vi "Idle_WeatherStationComms.vi"(0 "VISA in":refnum<visa-resource-name>="LuftWS", 5 "WS_Commands":enum16{"OpenWS", "ReadTRHP", "CloseWS"}(ring)=enum."ReadTRHP", 7 "wait (ms)":u32=50, 11 "Error In":errorcluster) -> (4 "VISA out":refnum<visa-resource-name>="LuftWS", 6 "TRHP":T1={"Temp"=27.834401709401718, "RelH"=23.501221001221, "Press"=837.9120879120879, "AbH"=6.333943833943834}, 8 "StringResponse":string, 15 "Error Out":errorcluster)   [LabVIEW 2012]
uses:
  WVD-MCSupdate/WVDNewArchitectureUpdate/WVD_Architecture_Update/WVDIAL_GlobalVariables.vi
  <vilib>/Instr/_visa.llb/VISA Configure Serial Port (Instr).vi
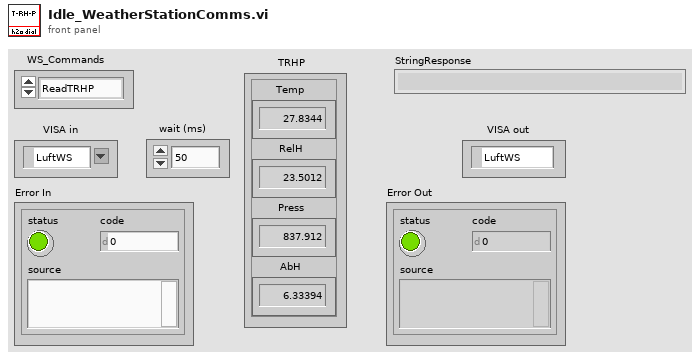
[diagram p1: front panel]
types:
  T1 = cluster{"Temp":dbl, "RelH":dbl, "Press":dbl, "AbH":dbl}
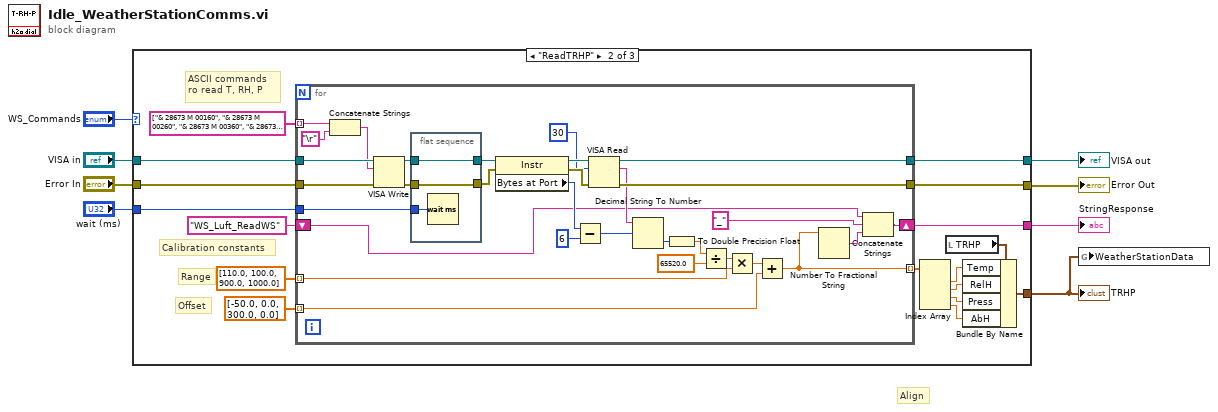
[diagram p0: block diagram]
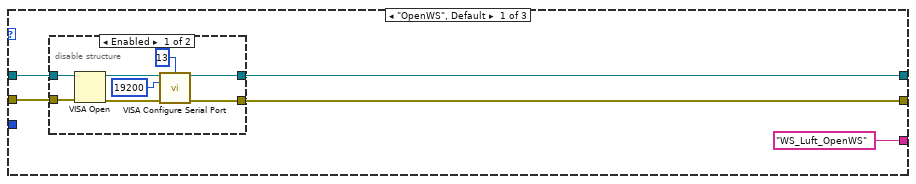
[diagram p2: hidden frame]
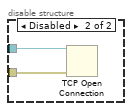
[diagram p3: hidden frame]
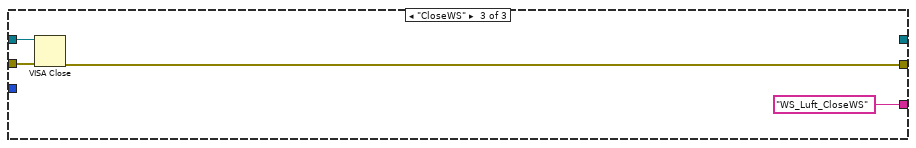
[diagram p4: hidden frame]
diagram:
  # "Align"
  n1 = case shown="\"ReadTRHP\"" "WS_Commands" {
    tunnel: "VISA in" -> [w13 w40 w78]
    tunnel: "Error In" -> [w12 w39 w77]
    tunnel: [w11 w37 _] -> w4
    tunnel: [w10 w36 w76] -> w3
    tunnel: "wait (ms)" -> [_ w38 _]
    tunnel: [_ w34 _] -> w2
    tunnel: ["WS_Luft_OpenWS" w25 "WS_Luft_CloseWS" ("String")] -> w1
    frame "OpenWS", Default {
      n2 = disable-structure shown="Enabled" {
        disable-tunnel: w13 -> [w19 w23]
        disable-tunnel: w12 -> [w18 w22]
        disable-tunnel: [w16 _] -> w11
        disable-tunnel: [w15 _] -> w10
        frame Enabled {
          n3 = VISA Open(error in (no error)=w18, VISA resource name=w19) -> (VISA resource name=w21:refnum<visa-resource-name>, error out=w17:errorcluster)  [unwired: 3 in]
          n4 = call-poly "VISA Configure Serial Port"("VISA resource name"=w21, "termination char\n(0xA = '\\n' = LF)"=u8 13 ("termination char\n(0xA = '\\n' = LF)"), "baud rate (9600)"=u32 19200, "error in (no error)"=w17) -> ("VISA resource name out"=w16:refnum<visa-resource-name>, "error out"=w15:errorcluster)  [unwired: 10 in]
        }
        frame Disabled {
          n5 = TCP Open Connection(address=w23, error in (no error)=w22) -> ()  [unwired: 3 in, 2 out]
        }
      }
    }
    frame "ReadTRHP" {
      # "Offset"
      # "Range"
      # "Calibration constants"
      # "ASCII commands\nro read T, RH, P"
      n6 = for {
        tunnel: w40 -> [w71]
        tunnel: w39 -> [w70]
        tunnel: w38 -> [w66]
        tunnel: [w61] -> w37
        tunnel: [w60] -> w36
        tunnel: [w41] -> w30 mode=indexing
        tunnel: string[] ["& 28673 M 00160", "& 28673 M 00260", "& 28673 M 00360", "& 28673 M 00270"] -> [w49] mode=indexing
        tunnel: dbl[] [110.0, 100.0, 900.0, 1000.0] -> [w48] mode=indexing
        tunnel: dbl[] [-50.0, 0.0, 300.0, 0.0] -> [w47] mode=indexing
        shift-right: [w44] -> w25
        shift-left: "WS_Luft_ReadWS" -> [w42]
        n7 = Concatenate Strings(w49, "\r") -> (w67:string)
        n8 = VISA Write(VISA resource name=w71, write buffer=w67, error in (no error)=w70) -> (VISA resource name out=w68:refnum<visa-resource-name>, error out=w69:errorcluster)  [unwired: 1 out]
        n9 = flat-sequence {
          tunnel: [w74] -> w63
          tunnel: w68 -> [w74]
          tunnel: [w73] -> w62
          tunnel: w69 -> [w73]
          tunnel: w66 -> [w72]
          frame #0 {
            n10 = Wait (ms)(milliseconds to wait=w72) -> ()  [unwired: 1 out]
          }
        }
        n11 = property class="Instr"(reference=w63, error in=w62) -> (reference out=w64:refnum<visa-resource-name>, error out=w65:errorcluster, "Bytes at Port"=w59:u32)
        n12 = Subtract(x=w59, y=u32 6) -> (x-y=w56:u32)
        n13 = VISA Read(VISA resource name=w64, byte count=u32 30, error in (no error)=w65) -> (VISA resource name out=w61:refnum<visa-resource-name>, read buffer=w57:string, error out=w60:errorcluster)  [unwired: 1 out]
        n14 = Decimal String To Number(string=w57, offset=w56) -> (number=w55:i32)  [unwired: 1 in, 1 out]
        n15 = To Double Precision Float(number=w55) -> (double precision float=w54:dbl)
        n16 = Divide(x=w54, y=65520.0) -> (x/y=w53:dbl)
        n17 = Multiply(x=w53, y=w48) -> (x*y=w52:dbl)
        n18 = Add(x=w52, y=w47) -> (x+y=w41:dbl)
        n19 = Number To Fractional String(number=w41) -> (F-format string=w45:string)  [unwired: 3 in]
        n20 = Concatenate Strings(w42, "_", w45) -> (w44:string)
      }
      n21 = Index Array(array=w30) -> (element #1=w27:dbl, element #2=w28:dbl, element #3=w29:dbl, element #4=w26:dbl)  [unwired: 4 in]
      n22 = local read "TRHP"() -> (w35:T1)
      n23 = Bundle By Name(cluster=w35, "Temp"=w27, "RelH"=w28, "Press"=w29, "AbH"=w26) -> (w34:T1)
    }
    frame "CloseWS" {
      n24 = VISA Close(VISA resource name=w78, error in (no error)=w77) -> (error out=w76:errorcluster)
    }
  }
  "Error Out" <- w3
  "VISA out" <- w4
  "TRHP" <- w2
  "StringResponse" <- w1
  n25 = global write "WVDIAL_GlobalVariables.vi" "WeatherStationData"(w2) -> ()
